vi "KnowPosition.vi"() -> ()   [LabVIEW 2018]
uses:
  outputs.vi
  refnums.vi
  sensors.vi
panel:
  out "Robot Position":cluster{dbl[], dbl[]}(graph)
  in  "Reset Positon":bool
  out "Heading (deg)":dbl format="%#_13g"
  out "Y Position (in)":dbl
  out "X Position (in)":dbl
  in  "Plot Data":bool
  out "Drive Encoder Velocities":cluster{dbl, dbl}
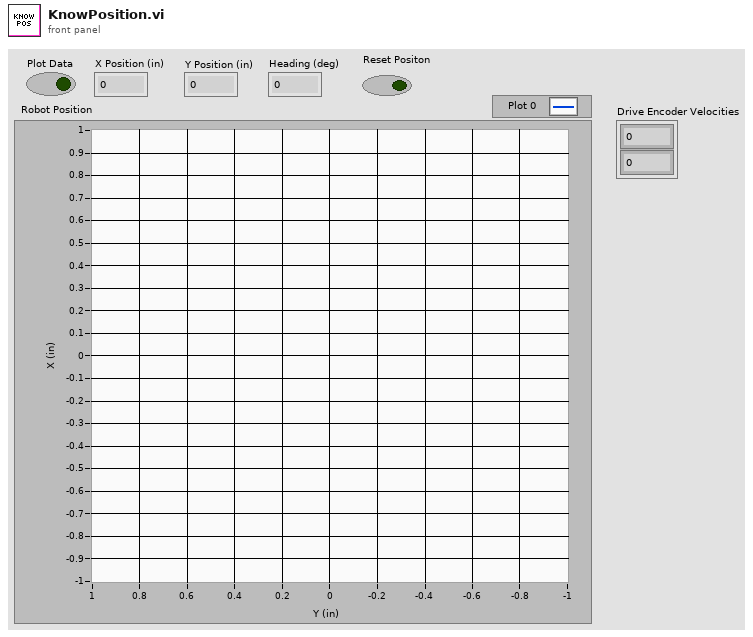
[diagram p1: front panel]
types:
  T1 = typedef "WPI_MotorControlDeviceRef.ctl" = cluster{"DeviceStatus":errorcluster, "Type":T2, "PWM":cluster{"PWM Channel":T3, "DeadBand":T4}, "CAN":cluster{"Device Number":u8, "SetOutput VI Ref":variant, "GetOutput VI Ref":variant, "Enable VI Ref":variant, "Disable VI Ref":variant, "Data":variant}, "Invert":bool, "DIO PWM":cluster{"PWM \"Enable\" Channel":T3, "DIOChannel":T5, "PWM Rate":dbl}}
  T2 = typedef "WPI_MotorControlType.ctl" = enum16{"PWM", "CAN", "DIO PWM"}
  T3 = typedef "FPGA_DIOPWMChannel.ctl" = enum8{"PWM 0", "PWM 1", "PWM 2", "PWM 3", "PWM 4", "PWM 5", "PWM 6", "PWM 7", "PWM 8", "PWM 9", "PWM MXP 0", "PWM MXP 1", "PWM MXP 2", "PWM MXP 3", "PWM MXP 4", "PWM MXP 5", "PWM MXP 6", "PWM MXP 7", "PWM MXP 8", "PWM MXP 9", "Invalid"}
  T4 = typedef "WPI_PWMDeadband.ctl" = cluster{"Name":string, "maxPositivePwm":i32, "minPositivePwm":i32, "centerPwm":i32, "maxNegativePwm":i32, "minNegativePwm":i32, "angularRange":u16}
  T5 = typedef "FPGA_DIOChannel.ctl" = enum8{"DIO 0", "DIO 1", "DIO 2", "DIO 3", "DIO 4", "DIO 5", "DIO 6", "DIO 7", "DIO 8", "DIO 9", "DIO MXP 0", "DIO MXP 1", "DIO MXP 2", "DIO MXP 3", "DIO MXP 4", "DIO MXP 5", "DIO MXP 6", "DIO MXP 7", "DIO MXP 8", "DIO MXP 9", "DIO MXP 10", "DIO MXP 11", "DIO MXP 12", "DIO MXP 13", "DIO MXP 14", "DIO MXP 15", "SPI Port CS1", "SPI Port CS2", "SPI Port CS3", "SPI Port MISO", "SPI Port MOSI", "Invalid"}
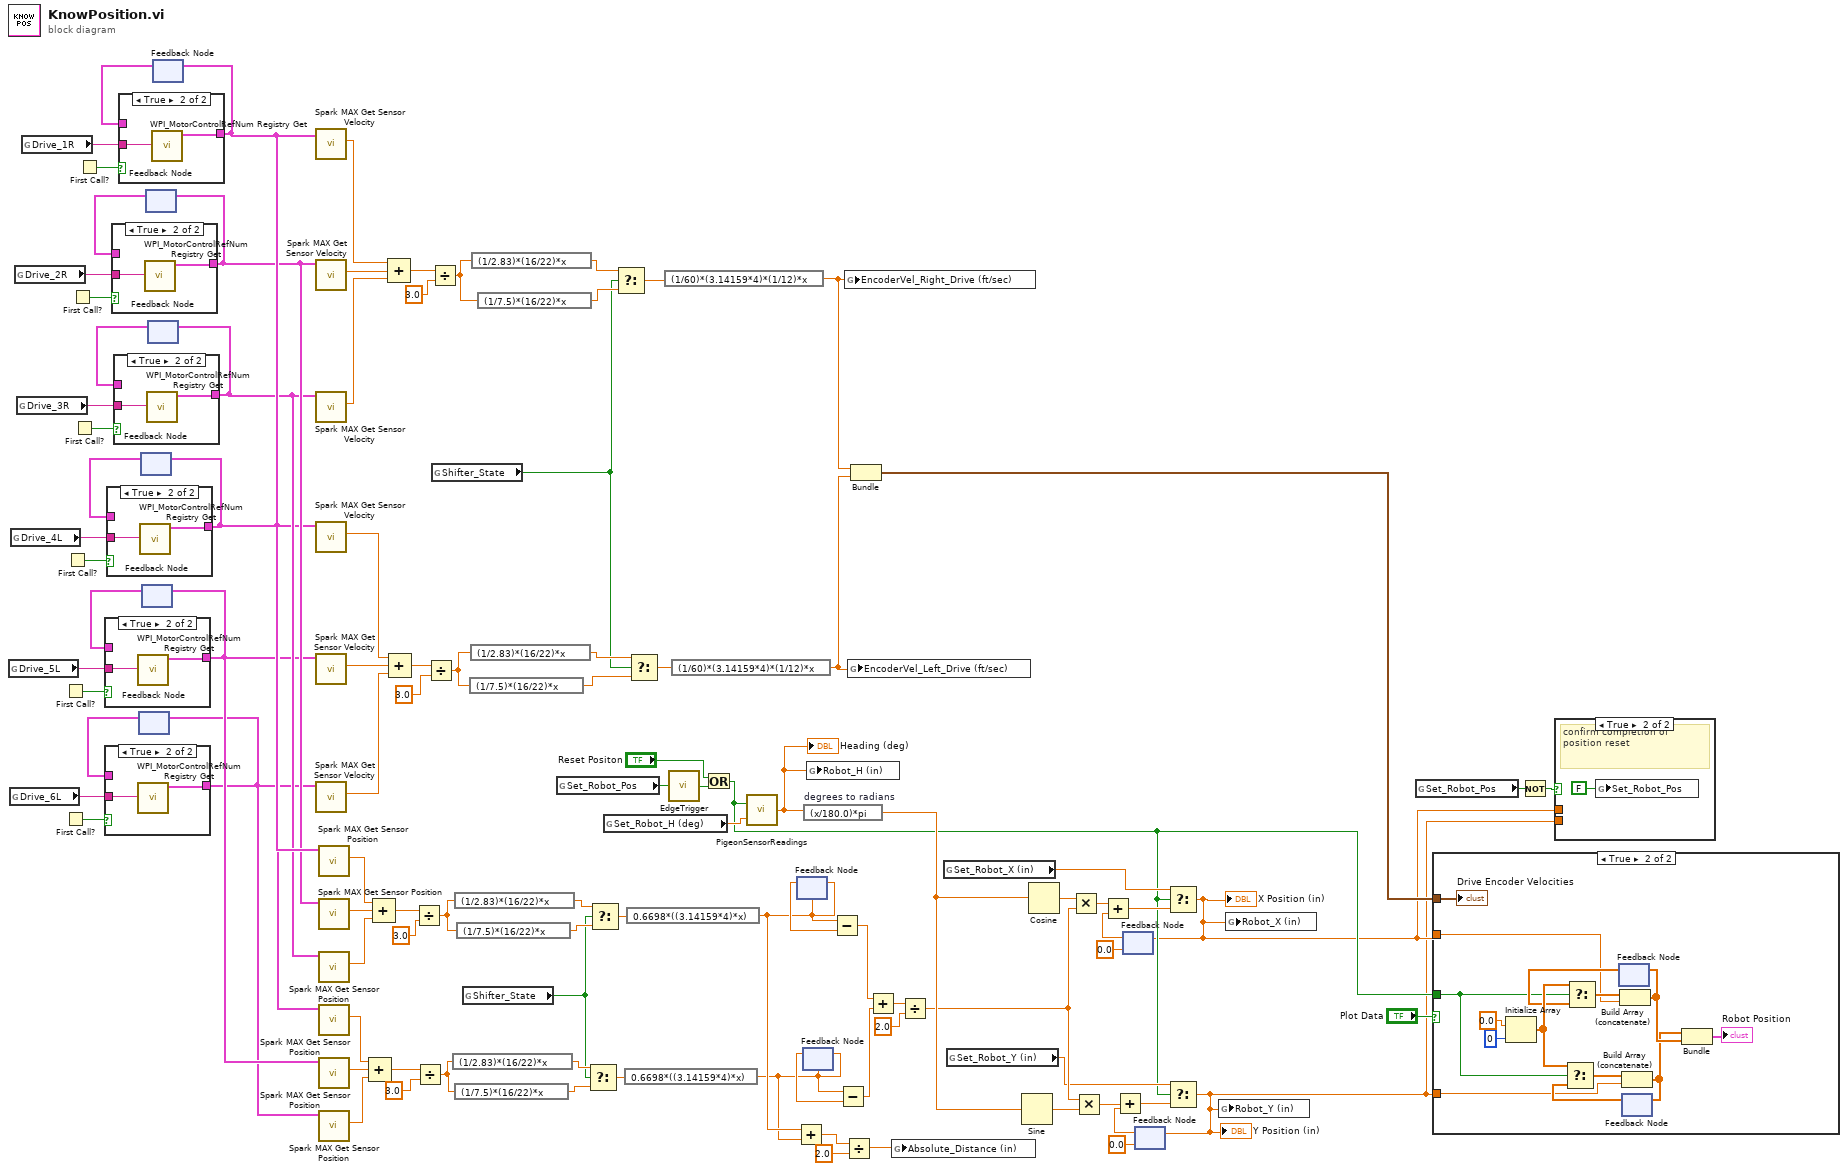
[diagram p0: block diagram]
diagram:
  n1 = global read "refnums.vi" "Drive_5L"() -> (w32:string)
  n2 = global read "refnums.vi" "Drive_6L"() -> (w28:string)
  n3 = global read "refnums.vi" "Drive_4L"() -> (w39:string)
  n4 = global read "refnums.vi" "Drive_2R"() -> (w45:string)
  n5 = global read "refnums.vi" "Drive_3R"() -> (w42:string)
  n6 = global read "refnums.vi" "Drive_1R"() -> (w48:string)
  n7 = First Call?() -> (First Call?: T/F=w34:bool)
  n8 = First Call?() -> (First Call?: T/F=w30:bool)
  n9 = First Call?() -> (First Call?: T/F=w41:bool)
  n10 = First Call?() -> (First Call?: T/F=w47:bool)
  n11 = First Call?() -> (First Call?: T/F=w44:bool)
  n12 = First Call?() -> (First Call?: T/F=w50:bool)
  n13 = feedback #1() -> (w29:T1)  [unwired: 1 in]
  n14 = case shown="True" w30 {
    tunnel: [w102 w103] -> w27
    tunnel: w29 -> [w102 _]
    tunnel: w28 -> [_ w104]
    frame False {
    }
    frame True {
      n15 = call <vilib>:"WPI_MotorControlRefNum Registry Get.vi"("refnum name"=w104) -> ("MotorControlDevRef"=w103:T1)  [unwired: 9 in, 1 out]
    }
  }
  n16 = feedback-in #1(w27) -> ()
  n17 = feedback #2() -> (w40:T1)  [unwired: 1 in]
  n18 = case shown="True" w41 {
    tunnel: [w105 w106] -> w35
    tunnel: w40 -> [w105 _]
    tunnel: w39 -> [_ w107]
    frame False {
    }
    frame True {
      n19 = call <vilib>:"WPI_MotorControlRefNum Registry Get.vi"("refnum name"=w107) -> ("MotorControlDevRef"=w106:T1)  [unwired: 9 in, 1 out]
    }
  }
  n20 = feedback-in #2(w35) -> ()
  n21 = feedback #3() -> (w33:T1)  [unwired: 1 in]
  n22 = case shown="True" w34 {
    tunnel: [w108 w109] -> w31
    tunnel: w33 -> [w108 _]
    tunnel: w32 -> [_ w110]
    frame False {
    }
    frame True {
      n23 = call <vilib>:"WPI_MotorControlRefNum Registry Get.vi"("refnum name"=w110) -> ("MotorControlDevRef"=w109:T1)  [unwired: 9 in, 1 out]
    }
  }
  n24 = feedback-in #3(w31) -> ()
  n25 = feedback #4() -> (w46:T1)  [unwired: 1 in]
  n26 = case shown="True" w47 {
    tunnel: [w111 w112] -> w37
    tunnel: w46 -> [w111 _]
    tunnel: w45 -> [_ w113]
    frame False {
    }
    frame True {
      n27 = call <vilib>:"WPI_MotorControlRefNum Registry Get.vi"("refnum name"=w113) -> ("MotorControlDevRef"=w112:T1)  [unwired: 9 in, 1 out]
    }
  }
  n28 = feedback-in #4(w37) -> ()
  n29 = feedback #5() -> (w43:T1)  [unwired: 1 in]
  n30 = case shown="True" w44 {
    tunnel: [w114 w115] -> w36
    tunnel: w43 -> [w114 _]
    tunnel: w42 -> [_ w116]
    frame False {
    }
    frame True {
      n31 = call <vilib>:"WPI_MotorControlRefNum Registry Get.vi"("refnum name"=w116) -> ("MotorControlDevRef"=w115:T1)  [unwired: 9 in, 1 out]
    }
  }
  n32 = feedback-in #5(w36) -> ()
  n33 = feedback #6() -> (w49:T1)  [unwired: 1 in]
  n34 = case shown="True" w50 {
    tunnel: [w117 w118] -> w38
    tunnel: w49 -> [w117 _]
    tunnel: w48 -> [_ w119]
    frame False {
    }
    frame True {
      n35 = call <vilib>:"WPI_MotorControlRefNum Registry Get.vi"("refnum name"=w119) -> ("MotorControlDevRef"=w118:T1)  [unwired: 9 in, 1 out]
    }
  }
  n36 = feedback-in #6(w38) -> ()
  n37 = call <vilib>:"Spark MAX Get Sensor Velocity.vi"("MotorControlDevRef in"=w38) -> ("Sensor Velocity"=w101:dbl)  [unwired: 7 in, 3 out]
  n38 = call <vilib>:"Spark MAX Get Sensor Velocity.vi"("MotorControlDevRef in"=w37) -> ("Sensor Velocity"=w100:dbl)  [unwired: 7 in, 3 out]
  n39 = call <vilib>:"Spark MAX Get Sensor Velocity.vi"("MotorControlDevRef in"=w36) -> ("Sensor Velocity"=w99:dbl)  [unwired: 7 in, 3 out]
  n40 = call <vilib>:"Spark MAX Get Sensor Velocity.vi"("MotorControlDevRef in"=w35) -> ("Sensor Velocity"=w98:dbl)  [unwired: 7 in, 3 out]
  n41 = call <vilib>:"Spark MAX Get Sensor Velocity.vi"("MotorControlDevRef in"=w31) -> ("Sensor Velocity"=w97:dbl)  [unwired: 7 in, 3 out]
  n42 = call <vilib>:"Spark MAX Get Sensor Velocity.vi"("MotorControlDevRef in"=w27) -> ("Sensor Velocity"=w96:dbl)  [unwired: 7 in, 3 out]
  n43 = call <vilib>:"Spark MAX Get Sensor Position.vi"("MotorControlDevRef in"=w38) -> ("Sensor Position"=w81:dbl)  [unwired: 7 in, 3 out]
  n44 = call <vilib>:"Spark MAX Get Sensor Position.vi"("MotorControlDevRef in"=w37) -> ("Sensor Position"=w80:dbl)  [unwired: 7 in, 3 out]
  n45 = call <vilib>:"Spark MAX Get Sensor Position.vi"("MotorControlDevRef in"=w36) -> ("Sensor Position"=w79:dbl)  [unwired: 7 in, 3 out]
  n46 = call <vilib>:"Spark MAX Get Sensor Position.vi"("MotorControlDevRef in"=w35) -> ("Sensor Position"=w74:dbl)  [unwired: 7 in, 3 out]
  n47 = call <vilib>:"Spark MAX Get Sensor Position.vi"("MotorControlDevRef in"=w31) -> ("Sensor Position"=w73:dbl)  [unwired: 7 in, 3 out]
  n48 = call <vilib>:"Spark MAX Get Sensor Position.vi"("MotorControlDevRef in"=w27) -> ("Sensor Position"=w72:dbl)  [unwired: 7 in, 3 out]
  n49 = Compound Arithmetic op=ADD(w74, w73, w72) -> (w76:dbl)
  n50 = Compound Arithmetic op=ADD(w81, w80, w79) -> (w78:dbl)
  n51 = Compound Arithmetic op=ADD(w101, w100, w99) -> (w93:dbl)
  n52 = Compound Arithmetic op=ADD(w98, w97, w96) -> (w92:dbl)
  n53 = Divide(x=w78, y=3.0) -> (x/y=w21:dbl)
  n54 = Divide(x=w76, y=3.0) -> (x/y=w17:dbl)
  n55 = Divide(x=w92, y=3.0) -> (x/y=w91:dbl)
  n56 = Divide(x=w93, y=3.0) -> (x/y=w90:dbl)
  n57 = global read "outputs.vi" "Shifter_State"() -> (w53:bool)
  n58 = expression code="(1/2.83)*(16/22)*x"(w17) -> (w16:dbl)
  n59 = expression code="(1/2.83)*(16/22)*x"(w21) -> (w60:dbl)
  n60 = expression code="(1/7.5)*(16/22)*x"(w17) -> (w19:dbl)
  n61 = expression code="(1/7.5)*(16/22)*x"(w21) -> (w59:dbl)
  n62 = global read "outputs.vi" "Shifter_State"() -> (w13:bool)
  n63 = expression code="(1/7.5)*(16/22)*x"(w91) -> (w86:dbl)
  n64 = expression code="(1/2.83)*(16/22)*x"(w91) -> (w87:dbl)
  n65 = expression code="(1/2.83)*(16/22)*x"(w90) -> (w89:dbl)
  n66 = expression code="(1/7.5)*(16/22)*x"(w90) -> (w88:dbl)
  n67 = global read "sensors.vi" "Set_Robot_Pos"() -> (w9:bool)
  n68 = Select(t=w16, s=w13, f=w19) -> (s? t:f=w18:dbl)
  n69 = Select(t=w60, s=w13, f=w59) -> (s? t:f=w54:dbl)
  n70 = global read "sensors.vi" "Set_Robot_H (deg)"() -> (w10:dbl)
  n71 = Select(t=w89, s=w53, f=w88) -> (s? t:f=w85:dbl)
  n72 = expression code="0.6698*((3.14159*4)*x)"(w18) -> (w15:dbl)
  n73 = expression code="0.6698*((3.14159*4)*x)"(w54) -> (w20:dbl)
  n74 = Select(t=w87, s=w53, f=w86) -> (s? t:f=w84:dbl)
  n75 = expression code="(1/60)*(3.14159*4)*(1/12)*x"(w85) -> (w51:dbl)
  n76 = call "EdgeTrigger.vi"("Input Signal"=w9) -> ("All Edge Trigger"=w8:bool)  [unwired: 2 out]
  n77 = expression code="(1/60)*(3.14159*4)*(1/12)*x"(w84) -> (w52:dbl)
  n78 = Or(x="Reset Positon", y=w8) -> (x .or. y?=w6:bool)
  n79 = call "PigeonSensorReadings.vi"("Reset Yaw (deg)"=w10, "Reset Yaw"=w6) -> ("Yaw (deg)"=w1:dbl)
  "Heading (deg)" <- w1
  n80 = Add(x=w20, y=w15) -> (x+y=w24:dbl)
  n81 = feedback-in #7(w20) -> ()
  n82 = feedback #7(w20) -> (w58:dbl)
  n83 = feedback #8(w15) -> (w57:dbl)
  n84 = feedback-in #8(w15) -> ()
  n85 = expression code="(x/180.0)*pi" "degrees to radians"(w1) -> (w61:dbl)
  n86 = global write "sensors.vi" "Robot_H (in)"(w1) -> ()
  n87 = Subtract(x=w20, y=w58) -> (x-y=w26:dbl)
  n88 = Subtract(x=w15, y=w57) -> (x-y=w25:dbl)
  n89 = Divide(x=w24, y=2.0) -> (x/y=w14:dbl)
  n90 = global write "sensors.vi" "EncoderVel_Right_Drive (ft/sec)"(w51) -> ()
  n91 = global write "sensors.vi" "EncoderVel_Left_Drive (ft/sec)"(w52) -> ()
  n92 = Bundle(w51, w52) -> (w82:cluster{dbl, dbl})  [unwired: 1 in]
  n93 = Add(x=w26, y=w25) -> (x+y=w71:dbl)
  n94 = global write "sensors.vi" "Absolute_Distance (in)"(w14) -> ()
  n95 = Divide(x=w71, y=2.0) -> (x/y=w22:dbl)
  n96 = global read "sensors.vi" "Set_Robot_X (in)"() -> (w12:dbl)
  n97 = global read "sensors.vi" "Set_Robot_Y (in)"() -> (w11:dbl)
  n98 = Sine(x=w61) -> (sin(x)=w68:dbl)
  n99 = Cosine(x=w61) -> (cos(x)=w69:dbl)
  n100 = Multiply(x=w69, y=w22) -> (x*y=w67:dbl)
  n101 = Multiply(x=w22, y=w68) -> (x*y=w65:dbl)
  n102 = feedback #9(0.0) -> (w66:dbl)
  n103 = Add(x=w67, y=w66) -> (x+y=w55:dbl)
  n104 = feedback #10(0.0) -> (w64:dbl)
  n105 = Add(x=w65, y=w64) -> (x+y=w56:dbl)
  n106 = Select(t=w12, s=w6, f=w55) -> (s? t:f=w3:dbl)
  "X Position (in)" <- w3
  n107 = feedback-in #9(w3) -> ()
  n108 = Select(t=w11, s=w6, f=w56) -> (s? t:f=w2:dbl)
  "Y Position (in)" <- w2
  n109 = feedback-in #10(w2) -> ()
  n110 = global write "sensors.vi" "Robot_Y (in)"(w2) -> ()
  n111 = global write "sensors.vi" "Robot_X (in)"(w3) -> ()
  n112 = global read "sensors.vi" "Set_Robot_Pos"() -> (w5:bool)
  n113 = case shown="True" "Plot Data" {
    tunnel: w82 -> [_ w133]
    tunnel: w6 -> [_ w120]
    tunnel: w3 -> [_ w123]
    tunnel: w2 -> [_ w122]
    frame False {
    }
    frame True {
      n114 = Initialize Array(0.0 ("element"), 0 ("dimension size")) -> (w132:dbl[])
      n115 = feedback #11() -> (w128:dbl[])  [unwired: 1 in]
      n116 = Select(t=w132, s=w120, f=w128) -> (s? t:f=w129:dbl[])
      n117 = Build Array (concatenate)(w129, w123) -> (w127:dbl[])
      n118 = feedback-in #11(w127) -> ()
      n119 = feedback #12() -> (w130:dbl[])  [unwired: 1 in]
      n120 = Select(t=w132, s=w120, f=w130) -> (s? t:f=w131:dbl[])
      n121 = Build Array (concatenate)(w131, w122) -> (w126:dbl[])
      n122 = feedback-in #12(w126) -> ()
      n123 = Bundle(w126, w127) -> (→"Robot Position":cluster{dbl[], dbl[]})  [unwired: 1 in]
      "Drive Encoder Velocities" <- w133
    }
  }
  n124 = Not(x=w5) -> (.not. x?=w4:bool)
  n125 = case shown="True" w4 {
    tunnel: w3 -> [_ _]
    tunnel: w2 -> [_ _]
    frame False {
    }
    frame True {
      # "confirm completion of position reset"
      n126 = global write "sensors.vi" "Set_Robot_Pos"(FALSE ("Set_Robot_Pos")) -> ()
    }
  }
